vi "Array streng monoton steigend.vi"(7 "Array":dbl[](array[numeric]) format="%_10g") -> (4 "Array 3":i32[](array[numeric]), 8 "Array 2":dbl[](array[numeric]))   [LabVIEW 2017, in "util.lvlib"]
uses:
  util.lvlib
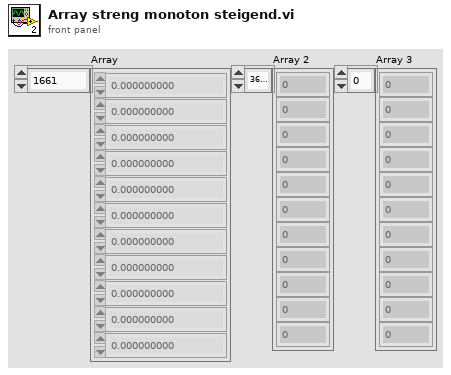
[diagram p1: front panel]
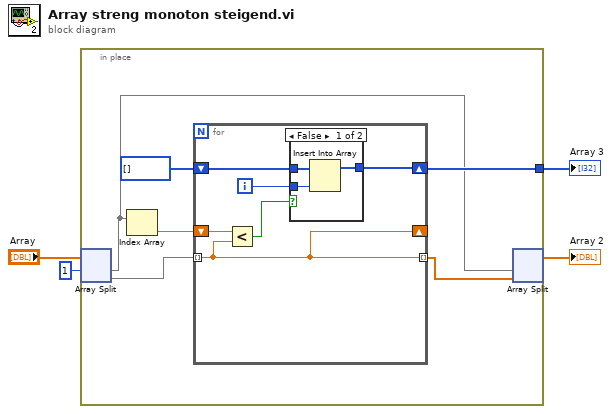
[diagram p0: block diagram]
diagram:
  n1 = in-place {
    in-place-border: [w9] -> w4
    n2 = in-place-split #1("Array", 1) -> (w5:dbl[], w8:dbl[])
    n3 = Index Array(array=w5) -> (element=w7:dbl)  [unwired: 1 in]
    n4 = for {
      tunnel: w8 -> [w12] mode=indexing
      shift-right: [w12] -> _
      shift-left: w7 -> [w16]
      shift-right: [w13] -> w9
      shift-left: i32[] [] -> [w11]
      tunnel: [w12] -> w6 mode=indexing
      i -> [w14]
      n5 = Less?(x=w16, y=w12) -> (x < y?=w15:bool)
      n6 = case shown="False" w15 {
        tunnel: w14 -> [w19 _]
        tunnel: [w18 w20] -> w13
        tunnel: w11 -> [w17 w20]
        frame False {
          n7 = Insert Into Array(array=w17, new element=w19) -> (w18:i32[])  [unwired: 1 in]
        }
        frame True {
        }
      }
    }
    n8 = in-place-split #1(w5, w6) -> (→"Array 2":dbl[])  [unwired: 1 out]
  }
  "Array 3" <- w4
